vi "Database.vi"(0 "Name":string, 1 "Action":enum16{"ClearUsers", "GetUsers", "AddUser"}(ring), 5 "Surname":string, 7 "Age":string, 9 "Nationality":string, 11 "error in":errorcluster) -> (4 "Users":string, 15 "error constant":errorcluster)   [LabVIEW 2022 SP3]
uses:
  1dd01c9a-6504-4094-adc1-cb5d036f8eff.vi
  <vilib>/Array/Sort 2D Array - Pop Stack.vi
  <vilib>/Array/Sort 2D Array - Push Stack.vi
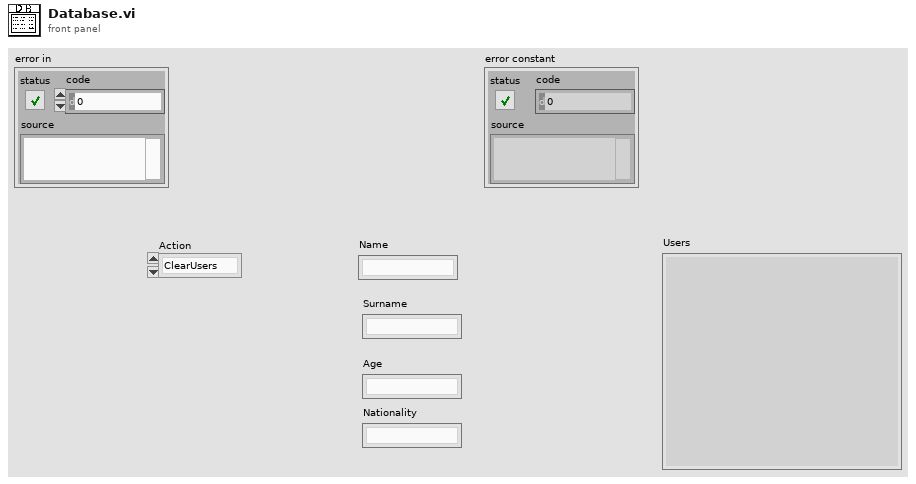
[diagram p1: front panel]
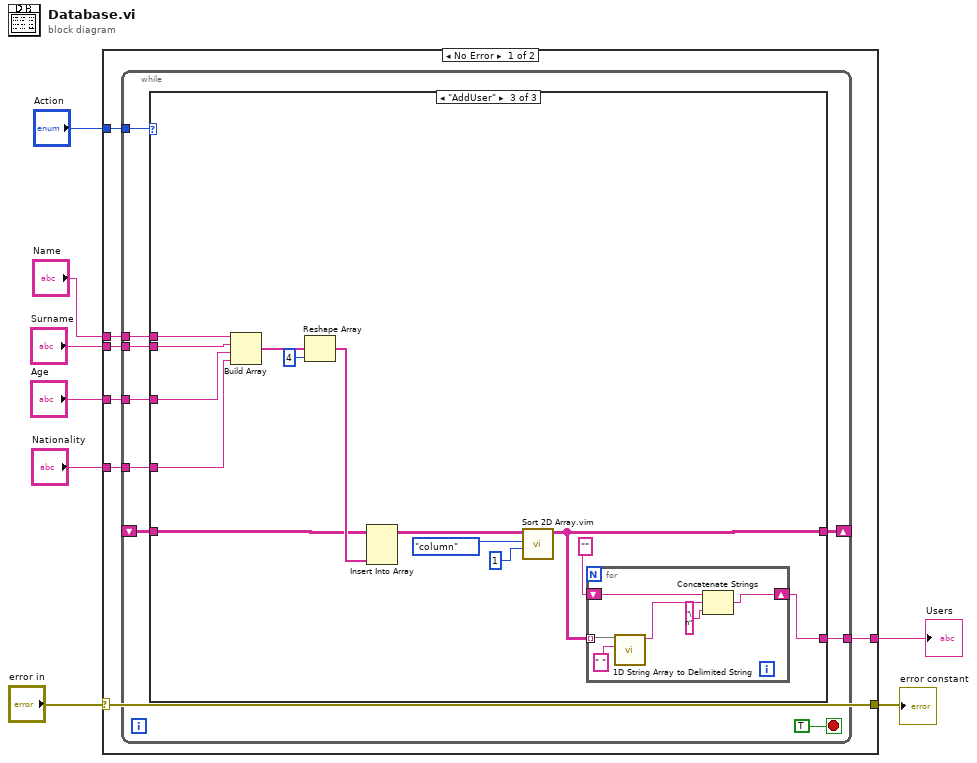
[diagram p0: block diagram]
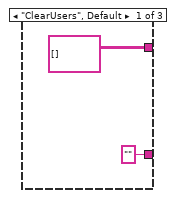
[diagram p2: hidden frame]
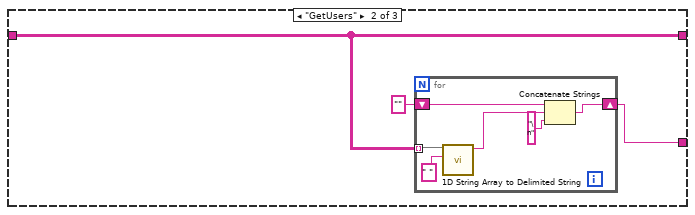
[diagram p3: hidden frame]
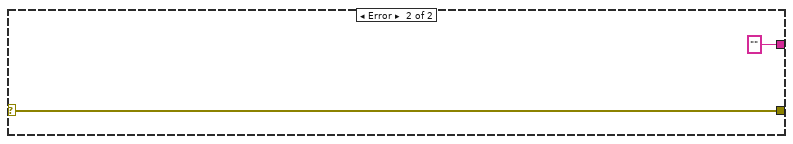
[diagram p4: hidden frame]
diagram:
  n1 = case shown="No Error" "error in" {
    selector: "error in" -> [w15 w57]
    tunnel: [w15 w57] -> w7
    tunnel: "Action" -> [w14 _]
    tunnel: [w9 "" ("delimited string")] -> w5
    tunnel: "Name" -> [w13 _]
    tunnel: "Surname" -> [w12 _]
    tunnel: "Age" -> [w11 _]
    tunnel: "Nationality" -> [w10 _]
    frame No Error {
      n2 = while {
        tunnel: w14 -> [w23]
        tunnel: w13 -> [w22]
        tunnel: w12 -> [w21]
        tunnel: w11 -> [w20]
        tunnel: w10 -> [w19]
        shift-right: [w17] -> _
        shift-left: _ -> [w18]
        tunnel: [w16] -> w9
        stop <- TRUE stop-if-true
        n3 = case shown="\"AddUser\"" w23 {
          tunnel: w22 -> [_ _ w49]
          tunnel: w21 -> [_ _ w48]
          tunnel: w20 -> [_ _ w47]
          tunnel: w19 -> [_ _ w46]
          tunnel: w18 -> [_ w28 w42]
          tunnel: [string[][] [] w28 w38] -> w17
          tunnel: ["" ("delimited string") w29 w36] -> w16
          frame "ClearUsers", Default {
          }
          frame "GetUsers" {
            n4 = for {
              tunnel: w28 -> [w35] mode=indexing
              shift-right: [w32] -> w29
              shift-left: "" -> [w33]
              n5 = call <vilib>:"1D String Array to Delimited String.vi"("delimiter"=" ", "string array"=w35) -> ("delimited string"=w31:string)  [unwired: 9 in]
              n6 = Concatenate Strings(w33, w31, "\n" ("string")) -> (w32:string)
            }
          }
          frame "AddUser" {
            n7 = Build Array(w49, w48, w47, w46) -> (w45:string[])
            n8 = Reshape Array(w45, 4 ("dimension size")) -> (w43:string[])
            n9 = Insert Into Array(array=w42, new element=w43) -> (w41:string[][])  [unwired: 2 in]
            n10 = call "Sort 2D Array.vim"("index"=1, "dimension to index (column)"=enum16{"column", "row"}."column", "2D array"=w41) -> ("sorted 2D array"=w38:string[][])  [unwired: 7 in, 1 out]
            n11 = for {
              tunnel: w38 -> [w55] mode=indexing
              shift-right: [w52] -> w36
              shift-left: "" -> [w53]
              n12 = call <vilib>:"1D String Array to Delimited String.vi"("delimiter"=" ", "string array"=w55) -> ("delimited string"=w51:string)  [unwired: 9 in]
              n13 = Concatenate Strings(w53, w51, "\n" ("string")) -> (w52:string)
            }
          }
        }
      }
    }
    frame Error {
    }
  }
  "Users" <- w5
  "error constant" <- w7
